vi "Check for Carpet.vi"(5 "Original Mask":T1, 7 "Original Color":T1, 8 "Carpet Colors":T3, 9 "Carpet Selector":T4(ring), 10 "Combine Carpet Mask":bool=TRUE, 11 "Initial Scores":T2(array[cluster])) -> (2 "Updated Mask":T1, 3 "Updated Scores":T2(array[cluster]))   [LabVIEW 2014]
doc: "Construct a rectangle below the bin, check for the appropriate color of carpet and update the score, possibly the mask for visual display."
uses:
  <vilib>/vision/Image Controls.llb/IMAQ Image.ctl
  <vilib>/vision/NI_Vision_Development_Module.lvlib
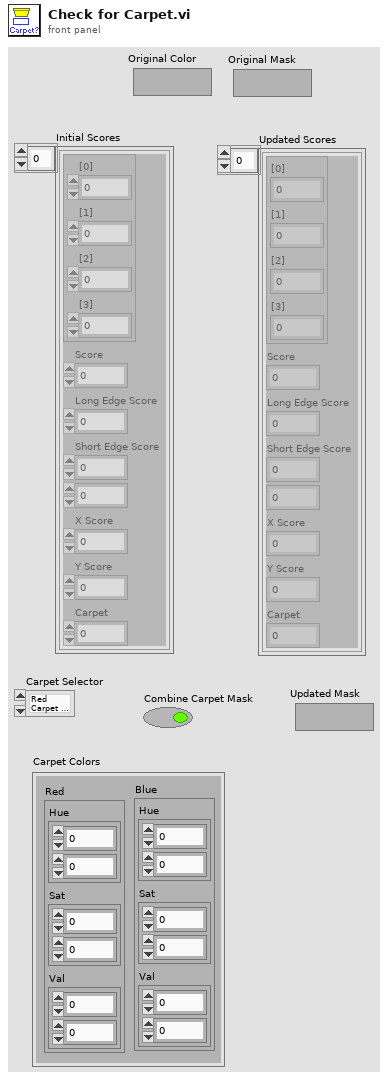
[diagram p1: front panel]
types:
  T1 = typedef "IMAQ Image.ctl" = refnum<image>
  T2 = cluster{cluster{"[0]":dbl, "[1]":dbl, "[2]":dbl, "[3]":dbl}, "Score":dbl, "Long Edge Score":dbl, "Short Edge Score":dbl, dbl, "X Score":dbl, "Y Score":dbl, "Carpet":dbl}[]
  T3 = cluster{"Red":cluster{"Hue":cluster{dbl, dbl}, "Sat":cluster{dbl, dbl}, "Val":cluster{dbl, dbl}}, "Blue":cluster{"Hue":cluster{dbl, dbl}, "Sat":cluster{dbl, dbl}, "Val":cluster{dbl, dbl}}}
  T4 = enum32{"Red Carpet Color", "Blue Carpet Color", "None"}
  T5 = typedef "Image Type" = u32
  T6 = cluster{"Hue":cluster{dbl, dbl}, "Sat":cluster{dbl, dbl}, "Val":cluster{dbl, dbl}}
  T7 = typedef "Particle Parameters" = i32
  T8 = cluster{"[0]":dbl, "[1]":dbl, "[2]":dbl, "[3]":dbl}
  T9 = cluster{cluster{"[0]":dbl, "[1]":dbl, "[2]":dbl, "[3]":dbl}, "Score":dbl, "Long Edge Score":dbl, "Short Edge Score":dbl, dbl, "X Score":dbl, "Y Score":dbl, "Carpet":dbl}
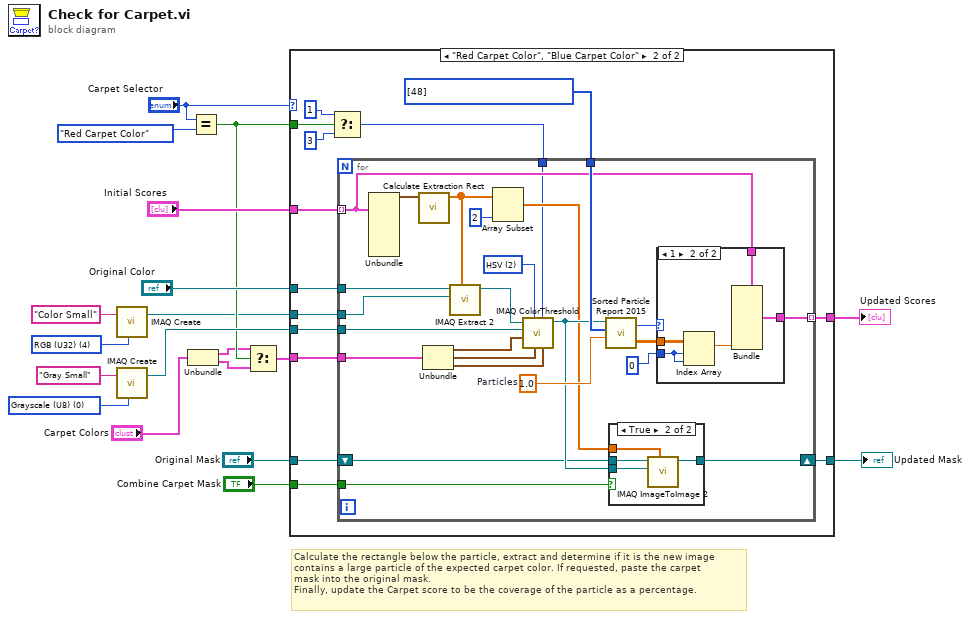
[diagram p0: block diagram]
diagram:
  w16 = T5 0 items=["Grayscale (U8)", "Grayscale (I16)", "Grayscale (SGL)", "Complex (CSG)", "RGB (U32)", "HSL (U32)", "RGB (U64)", "Grayscale (U16)"] ("Image Type")
  w13 = T5 4 items=["Grayscale (U8)", "Grayscale (I16)", "Grayscale (SGL)", "Complex (CSG)", "RGB (U32)", "HSL (U32)", "RGB (U64)", "Grayscale (U16)"] ("Image Type")
  # "Calculate the rectangle below the particle, extract and determine if it is the new image\ncontains a large particle of the expected carpet color. If requested, paste the carpet\nmask into the original mask.\nFinally, update the Carpet score to be the coverage of the particle as a percentage."
  n1 = call "IMAQ Create"("Image Name"="Color Small", "Image Type"=w13) -> ("New Image"=w5:T1)  [unwired: 2 in, 2 out]
  n2 = call "IMAQ Create"("Image Name"="Gray Small", "Image Type"=w16) -> ("New Image"=w12:T1)  [unwired: 2 in, 2 out]
  n3 = Unbundle("Carpet Colors") -> ("Red"=w3:T6, "Blue"=w2:T6)
  n4 = Equal?(x="Carpet Selector", y=T4."Red Carpet Color" ("Carpet Selector")) -> (x = y?=w6:bool)
  n5 = Select(t=w3, s=w6, f=w2) -> (s? t:f=w1:T6)
  n6 = case shown="\"Red Carpet Color\", \"Blue Carpet Color\"" "Carpet Selector" {
    tunnel: "Initial Scores" -> [w21 w35]
    tunnel: w1 -> [_ w34]
    tunnel: w12 -> [_ w33]
    tunnel: [w21 w31] -> w18
    tunnel: "Original Color" -> [_ w30]
    tunnel: "Combine Carpet Mask" -> [_ w29]
    tunnel: "Original Mask" -> [w20 w28]
    tunnel: [w20 w27] -> w9
    tunnel: w6 -> [_ w26]
    tunnel: w5 -> [_ w22]
    frame "None", Default {
    }
    frame "Red Carpet Color", "Blue Carpet Color" {
      w32 = T7[] [48] items=["Center of Mass X", "Center of Mass Y", "First Pixel X", "First Pixel Y", "Bounding Rect Left", "Bounding Rect Top", "Bounding Rect Right", "Bounding Rect Bottom", "Max Feret Diameter Start X", "Max Feret Diameter Start Y", "Max Feret Diameter End X", "Max Feret Diameter End Y", "Max Horiz. Segment Length Left", "Max Horiz. Segment Length Right", "Max Horiz. Segment Length Row", "-", "Bounding Rect Width", "Bounding Rect Height", "Bounding Rect Diagonal", "Perimeter", "Convex Hull Perimeter", "Holes' Perimeter", "Max Feret Diameter", "Equivalent Ellipse Major Axis", "Equivalent Ellipse Minor Axis", "Equivalent Ellipse Minor Axis (Feret)", "Equivalent Rect Long Side", "Equivalent Rect Short Side", "Equivalent Rect Diagonal", "Equivalent Rect Short Side (Feret)", "Average Horiz. Segment Length", "Average Vert. Segment Length", "Hydraulic Radius", "Waddel Disk Diameter", "-", "Area", "Holes' Area", "Particle & Holes' Area", "Convex Hull Area", "Image Area", "-", "Number of Holes", "Number of Horiz. Segments", "Number of Vert. Segments", "-", "Orientation", "Max Feret Diameter Orientation", "-", "% Area/Image Area", "% Area/(Particle & Holes' Area)", "Ratio of Equivalent Ellipse Axes", "Ratio of Equivalent Rect Sides", "-", "Elongation Factor", "Compactness Factor", "Heywood Circularity Factor", "Type Factor", "-", "Sum X", "Sum Y", "Sum XX", "Sum XY", "Sum YY", "Sum XXX", "Sum XXY", "Sum XYY", "Sum YYY", "-", "Moment of Inertia XX", "Moment of Inertia XY", "Moment of Inertia YY", "Moment of Inertia XXX", "Moment of Inertia XXY", "Moment of Inertia XYY", "Moment of Inertia YYY", "Norm. Moment of Inertia XX", "Norm. Moment of Inertia XY", "Norm. Moment of Inertia YY", "Norm. Moment of Inertia XXX", "Norm. Moment of Inertia XXY", "Norm. Moment of Inertia XYY", "Norm. Moment of Inertia YYY", "Hu Moment 1", "Hu Moment 2", "Hu Moment 3", "Hu Moment 4", "Hu Moment 5", "Hu Moment 6", "Hu Moment 7"] ("Pixel Measurements")
      n7 = Select(t=1, s=w26, f=3) -> (s? t:f=w23:i32)
      n8 = for {
        tunnel: w30 -> [w60]
        tunnel: w35 -> [w47] mode=indexing
        tunnel: w34 -> [w58]
        tunnel: w33 -> [w54]
        tunnel: w32 -> [w52]
        tunnel: [w46] -> w31 mode=indexing
        tunnel: w29 -> [w45]
        shift-right: [w38] -> w27
        shift-left: w28 -> [w43]
        tunnel: w23 -> [w37]
        tunnel: w22 -> [w36]
        w51 = 1.0  # Particles
        w53 = u16 2 items=["RGB", "HSL", "HSV", "HSI"] ("Color Mode")
        n9 = Unbundle(w47) -> (w42:T8)  [unwired: 7 out]
        n10 = call "Calculate Extraction Rect.vi"("Particle Rect"=w42) -> ("Test Rect"=w39:dbl[])  [unwired: 10 in]
        n11 = Unbundle(w58) -> ("Hue"=w57:cluster{dbl, dbl}, "Sat"=w56:cluster{dbl, dbl}, "Val"=w55:cluster{dbl, dbl})
        n12 = call "IMAQ Extract 2"("Optional Rectangle"=w39, "Image Dst"=w36, "Image Src"=w60) -> ("Image Dst Out"=w59:T1)  [unwired: 7 in, 1 out]
        n13 = Array Subset(array=w39, length=2) -> (w41:dbl[])  [unwired: 1 in]
        n14 = call "IMAQ ColorThreshold"("Blue or Luma or Val or Inten Range"=w55, "Replace Value"=w37, "Green or Sat Range"=w56, "Color Mode"=w53, "Red or Hue Range"=w57, "Image Dst"=w54, "Image Src"=w59) -> ("Image Dst Out"=w44:T1)  [unwired: 3 in, 1 out]
        n15 = call "Sorted Particle Report 2015.vi"("Particle Count Limit"=w51, "Pixel Measurements"=w52, "Image in"=w44) -> ("Sorted Data"=w49:dbl[][], "Particles"=w50:i32)  [unwired: 1 in]
        n16 = case shown="True" w45 {
          tunnel: w44 -> [_ w65]
          tunnel: w43 -> [w61 w64]
          tunnel: w41 -> [_ w63]
          tunnel: [w61 w62] -> w38
          frame False {
          }
          frame True {
            n17 = call "IMAQ ImageToImage 2"("Offset Left/Top"=w63, "Image Src (Small)"=w65, "Image Src (Large)"=w64) -> ("Image Dst Out"=w62:T1)  [unwired: 7 in, 1 out]
          }
        }
        n18 = case shown="1" w50 {
          tunnel: w49 -> [_ w71]
          tunnel: 0 -> [_ w70]
          tunnel: w47 -> [w66 w69]
          tunnel: [w66 w67] -> w46
          frame 0, Default {
          }
          frame 1 {
            n19 = Index Array(array=w71, index (row)=w70, index (col)=w70) -> (element=w68:dbl)
            n20 = Bundle(cluster=w69, "Carpet"=w68) -> (w67:T9)  [unwired: 7 in]
          }
        }
      }
    }
  }
  "Updated Scores" <- w18
  "Updated Mask" <- w9
